vi "Load GaGe Hardware.vi"(8 "error in (no error)":errorcluster, 11 "vi path":path=path "C:/ProjectLocker/NHMFL/LANL/Libraries/GaGe-DAQ/Gage llb/GaGeListDevices.vi") -> (0 "error out":errorcluster, 3 "GaGe Devices":refnum<class "Mag Lab Hardware.lvclass">[](array[class]))   [LabVIEW 2015]
uses:
  Mag Lab Measure/Hardware/Mag Lab Hardware.lvclass
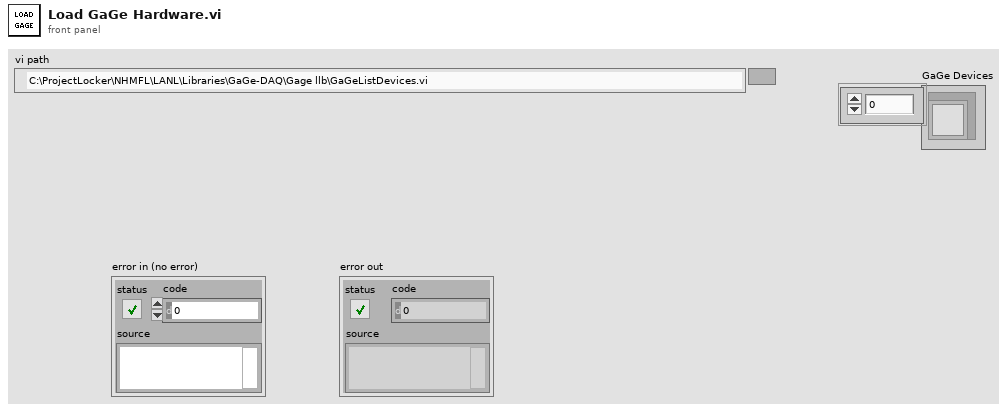
[diagram p1: front panel]
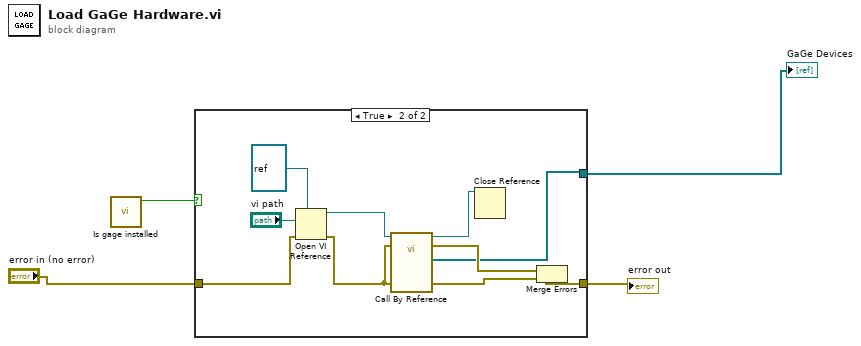
[diagram p0: block diagram]
diagram:
  n1 = call "Is gage installed.vi"() -> ("file or folder exists?"=w4:bool)  [unwired: 11 in]
  n2 = case shown="True" w4 {
    tunnel: "error in (no error)" -> [w5 w11]
    tunnel: [w5 w9] -> w2
    tunnel: [_ w7] -> w1
    frame False {
    }
    frame True {
      n3 = Open VI Reference(type specifier VI Refnum (for type only)=refnum<vi> refnum, vi path="vi path", error in (no error)=w11) -> (vi reference=w14:refnum<vi>, error out=w10:errorcluster)  [unwired: 3 in]
      n4 = call-by-ref "?"(reference=w14, error in=w10, "Error In"=w10) -> (reference out=w6:refnum<vi>, error out=w8:errorcluster, "Error Out"=w12:errorcluster, "GaGe Devices"=w7:refnum<class "Mag Lab Hardware.lvclass">[])  [unwired: 9 in]
      n5 = Close Reference(reference=w6) -> ()  [unwired: 1 in, 1 out]
      n6 = Merge Errors(w8, w12) -> (w9:errorcluster)
    }
  }
  "error out" <- w2
  "GaGe Devices" <- w1
